vi "Index Coincident Pairs.vi"(2 "Interpolation method":T1={"Mode"=enum."Interpolate", "Index"=[]}, 3 "Time Cluster 1":T2) -> (1 "Time Cluster 1 Out":T2)   [LabVIEW 2022 SP3]
uses:
  Controls/Time_Trace_Cluster.ctl
  Controls/Resample mode.ctl
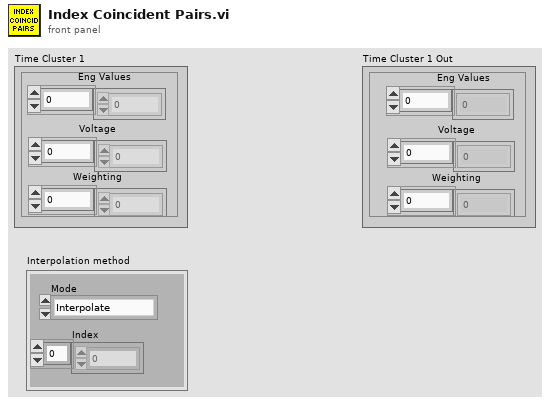
[diagram p1: front panel]
types:
  T1 = typedef "Resample mode.ctl" = cluster{"Mode":enum16{"Index", "Interpolate"}, "Index":dbl[]}
  T2 = typedef "Time_Trace_Cluster.ctl" = cluster{"Weighting":dbl[], "Voltage":dbl[], "Eng Values":dbl[]}
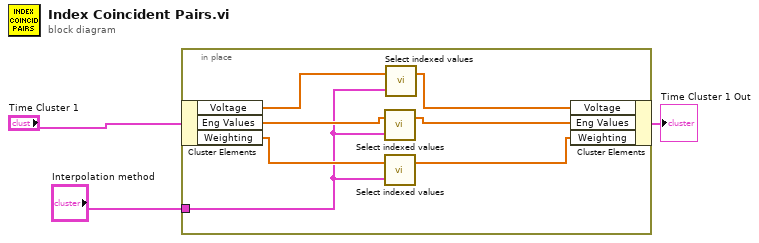
[diagram p0: block diagram]
diagram:
  n1 = in-place {
    in-place-border: "Interpolation method" -> [w7]
    n2 = in-place-cluster #1("Time Cluster 1") -> ("Voltage"=w10:dbl[], "Eng Values"=w9:dbl[], "Weighting"=w8:dbl[])
    n3 = call "Select indexed values.vi"("Cluster"=w7, "Values"=w9) -> ("Values Out"=w5:dbl[])  [unwired: 1 in]
    n4 = call "Select indexed values.vi"("Cluster"=w7, "Values"=w8) -> ("Values Out"=w4:dbl[])  [unwired: 1 in]
    n5 = call "Select indexed values.vi"("Cluster"=w7, "Values"=w10) -> ("Values Out"=w6:dbl[])  [unwired: 1 in]
    n6 = in-place-cluster #1("Voltage"=w6, "Eng Values"=w5, "Weighting"=w4) -> (→"Time Cluster 1 Out":T2)
  }
